vi "WriteU64ToU16FIFO.vi"(1 "U64":u64) -> ()   [LabVIEW 2016]
uses:
  <vilib>/rvi/interface/RandomDataEmulation/niFpgaRandomDataHandleErrors.vi
  <vilib>/rvi/DataTransferAndStorage/Container/Common/niFpgaContainerExecOnDevCompGetState.vi
  <vilib>/rvi/Emulation/niFpgaEmulationIsFPGAContextNoSignature.vi
  <vilib>/rvi/Emulation/niFpgaSctlEmulationGetInTimedLoop.vi
  <vilib>/rvi/errors/niFpgaSetErrorForExecOnDevCompSimple.vi
  <vilib>/rvi/eio/common/nirviEmuReportErrorAndStop.vi
  <vilib>/rvi/DataTransferAndStorage/Container/Common/niFpgaContainerGetUniqueNameForEmu.vi
  <vilib>/rvi/FIFO/Fifo_Resource/nirvififoEmulationSetSize.vi
  <vilib>/rvi/FIFO/Fifo_Resource/nirviFifoEmulationQueueMgr.vi
  <instcachedir>/0/nirviFifoEmulationQueueMgr_E5CAEC123FF24DC58D834DCA3CDAA9B5.lvgen/nirviFifoEmulationQueueMgr_E5CAEC123FF24DC58D834DCA3CDAA9B5_002.vi
  <vilib>/rvi/FIFO/Fifo_Resource/nirvififoEmulationDetermineInputValidOut.vi
  <vilib>/rvi/FIFO/Fifo_Resource/nirvififoEmulationCreateLock.vi
  <vilib>/rvi/Emulation/niFpgaProcessEmulError.vi
  <vilib>/rvi/FIFO/Fifo_Resource/nirvififoEmulationObtainLock.vi
  <vilib>/rvi/FIFO/Fifo_Resource/nirvififoEmulationReleaseLock.vi
  <vilib>/rvi/occurrence/nirviWaitOnOccurrenceBase.vi
  <vilib>/rvi/errors/nirviReportUnexpectedCaseInternalError.vi
  <vilib>/rvi/errors/nirviReportUnexpectedCaseInternalError (U32).vi
  <vilib>/Utility/error.llb/Clear Errors.vi
  <vilib>/rvi/DataTransferAndStorage/Container/XNode/niFpgaContainer.xnode
  <vilib>/rvi/interface/RandomDataEmulation/nirviRandomDataFpgaReadWriteTemplate.vi
  <vilib>/rvi/FIFO/Fifo_Resource/niFpgaFifoEmulationRefIn.vi
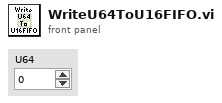
[diagram p1: front panel]
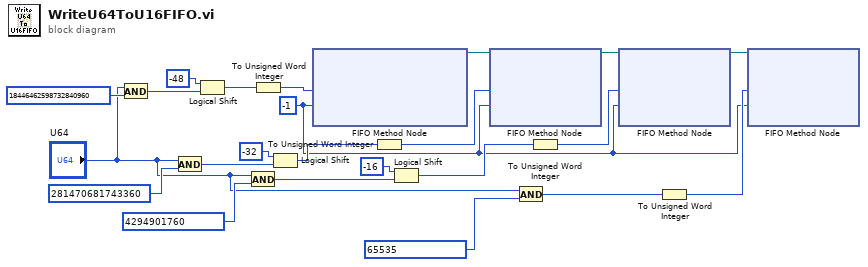
[diagram p0: block diagram]
diagram:
  w5 = -1 ("Timeout")
  n1 = And(x="U64", y=u64 18446462598732840960) -> (x .and. y?=w15:u64)
  n2 = And(x="U64", y=u64 281470681743360) -> (x .and. y?=w18:u64)
  n3 = Logical Shift(y=i16 -48, x=w15) -> (x << y=w13:u64)
  n4 = And(x="U64", y=u64 4294901760) -> (x .and. y?=w19:u64)
  n5 = To Unsigned Word Integer(number=w13) -> (unsigned 16bit integer=w10:u16)
  n6 = Logical Shift(y=i16 -32, x=w18) -> (x << y=w12:u64)
  n7 = xnode ("FIFO Method Node")("Element"=w10, "Timeout"=w5) -> ("FIFO Out"=w4:refnum<k21>)  [unwired: 1 in, 1 out]
  n8 = To Unsigned Word Integer(number=w12) -> (unsigned 16bit integer=w9:u16)
  n9 = Logical Shift(y=i16 -16, x=w19) -> (x << y=w11:u64)
  n10 = xnode ("FIFO Method Node")("Element"=w9, "Timeout"=w5, "FIFO In"=w4) -> ("FIFO Out"=w3:refnum<k21>)  [unwired: 1 out]
  n11 = And(x="U64", y=u64 65535) -> (x .and. y?=w20:u64)
  n12 = To Unsigned Word Integer(number=w11) -> (unsigned 16bit integer=w8:u16)
  n13 = xnode ("FIFO Method Node")("Element"=w8, "Timeout"=w5, "FIFO In"=w3) -> ("FIFO Out"=w2:refnum<k21>)  [unwired: 1 out]
  n14 = To Unsigned Word Integer(number=w20) -> (unsigned 16bit integer=w7:u16)
  n15 = xnode ("FIFO Method Node")("Element"=w7, "Timeout"=w5, "FIFO In"=w2) -> ()  [unwired: 2 out]
